vi "Check Local Formula Validity.vi"(7 "Fornula":string, 13 "Formula Interpreter's Path":path) -> (8 "Error?":bool)   [LabVIEW 2021, in "Formula.lvlib"]
uses:
  Formula.lvlib
  <vilib>/gmath/NI_Gmath.lvlib
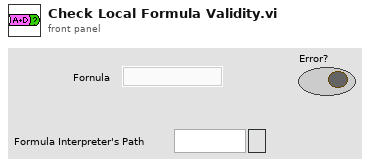
[diagram p1: front panel]
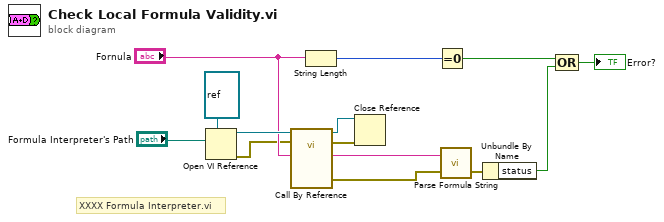
[diagram p0: block diagram]
diagram:
  # "XXXX Formula Interpreter.vi"
  n1 = Open VI Reference(type specifier VI Refnum (for type only)=refnum<vi> refnum, vi path="Formula Interpreter's Path") -> (vi reference=w9:refnum<vi>, error out=w5:errorcluster)  [unwired: 4 in]
  n2 = call-by-ref "?"(reference=w9, error in=w5, "Original Formula"="Fornula") -> (reference out=w2:refnum<vi>, error out=w3:errorcluster, 0:"error out"=w1:errorcluster, "Interpreted Formula"=w4:string)  [unwired: 6 in, 3 out]
  n3 = String Length(string="Fornula") -> (length=w11:i32)
  n4 = Close Reference(reference=w2, error in (no error)=w3) -> ()  [unwired: 1 out]
  n5 = Equal To 0?(x=w11) -> (x = 0?=w12:bool)
  n6 = call <vilib>:"Parse Formula String.vi"("error in (no error)"=w1, "formula"=w4) -> ("error out"=w10:errorcluster)  [unwired: 1 out]
  n7 = Unbundle By Name(w10) -> ("status"=w13:bool)
  n8 = Compound Arithmetic op=OR(w12, w13) -> (→"Error?":bool)
